vi "1TableHeaderPrefixDecoder.vi"(6 "ArrayIndex":i32, 8 "error in":errorcluster, 9 "Array?":bool, 10 "Added HeaderPrefix":string, 11 "Existing HeaderPrefix":string) -> (0 "error out":errorcluster, 3 "HeaderPrefix":string)   [LabVIEW 2014, in "TableLogger_Actor.lvlib" / "TableLogger_Actor.lvclass"]
uses:
  TableLogger_Actor.lvclass
panel:
  # "Connector Pane"
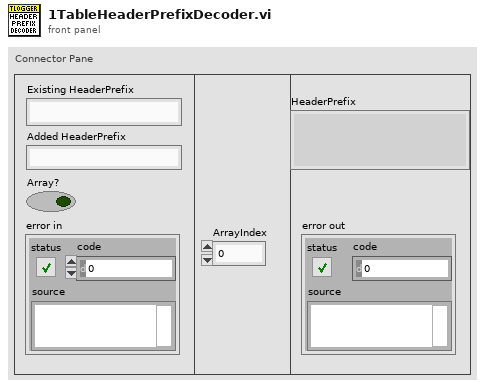
[diagram p1: front panel]
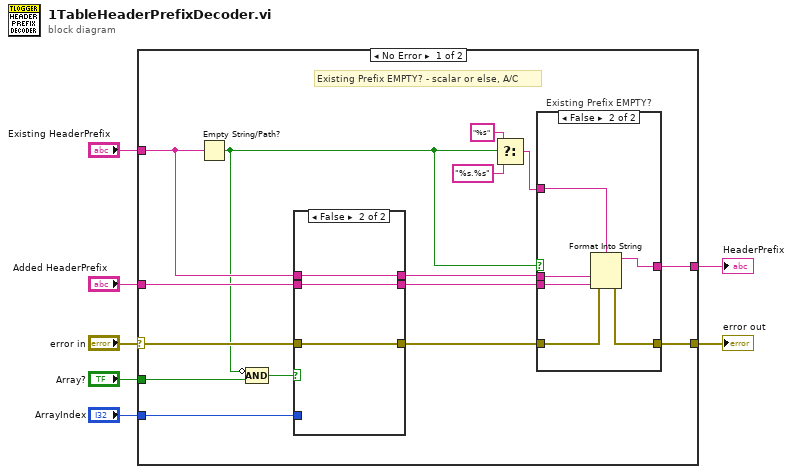
[diagram p0: block diagram]
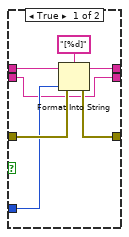
[diagram p2: hidden frame]
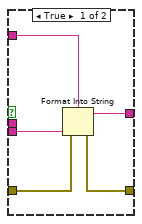
[diagram p3: hidden frame]
diagram:
  n1 = case shown="No Error" "error in" {
    selector: "error in" -> [w16 w44]
    tunnel: [w22 w44] -> w6
    tunnel: "Array?" -> [w21 _]
    tunnel: "Existing HeaderPrefix" -> [w17 _]
    tunnel: "ArrayIndex" -> [w20 _]
    tunnel: "Added HeaderPrefix" -> [w19 _]
    tunnel: [w18 _] -> w1
    frame No Error {
      # "Existing Prefix EMPTY? - scalar or else, A/C"
      n2 = Empty String/Path?(string/path=w17) -> (empty?=w10:bool)
      n3 = Compound Arithmetic op=AND(invert w10, w21) -> (w11:bool)
      n4 = case shown="False" w11 {
        tunnel: w16 -> [w29 w32]
        tunnel: [w28 w32] -> w12
        tunnel: w20 -> [w26 _]
        tunnel: [w25 w31] -> w9
        tunnel: w17 -> [w24 w31]
        tunnel: [w23 w30] -> w8
        tunnel: w19 -> [w23 w30]
        frame True {
          n5 = Format Into String(format string="[%d]", initial string=w24, error in=w29, w26) -> (resulting string=w25:string, error out=w28:errorcluster)
        }
        frame False {
        }
      }
      n6 = Select(t="%s" ("format string"), s=w10, f="%s.%s" ("format string")) -> (s? t:f=w13:string)
      n7 = case "Existing Prefix EMPTY?" shown="False" w10 {
        tunnel: w13 -> [w37 w43]
        tunnel: w8 -> [w36 w42]
        tunnel: [w35 w41] -> w18
        tunnel: w12 -> [w34 w40]
        tunnel: [w33 w39] -> w22
        tunnel: w9 -> [_ w38]
        frame True {
          n8 = Format Into String(format string=w37, error in=w34, w36) -> (resulting string=w35:string, error out=w33:errorcluster)  [unwired: 1 in]
        }
        frame False {
          n9 = Format Into String(format string=w43, error in=w40, w38, w42) -> (resulting string=w41:string, error out=w39:errorcluster)  [unwired: 1 in]
        }
      }
    }
    frame Error {
    }
  }
  "HeaderPrefix" <- w1
  "error out" <- w6
